vi "String Destroy.vi"(8 "error in (no error)":errorcluster, 11 "String DVR in":refnum<data-value>) -> (0 "error out":errorcluster)   [LabVIEW 2010, in "MDSplus.lvlib"]
uses:
  <vilib>/MDSplus/Library/MDSplus.lvlib
  <vilib>/MDSplus/Classes/Data_Class/Scalar_Class/String_Class/String.lvclass
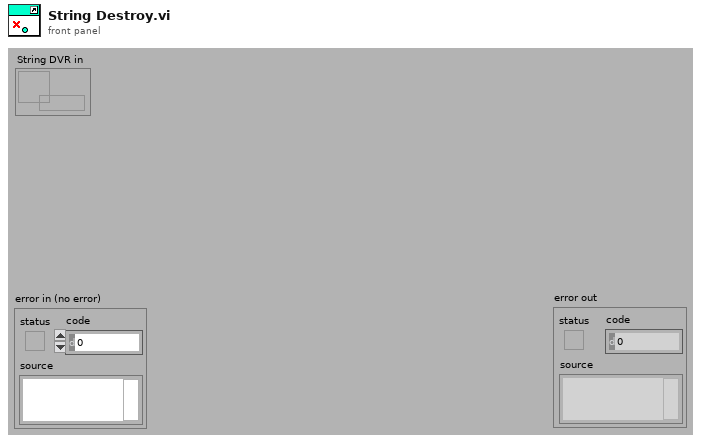
[diagram p1: front panel]
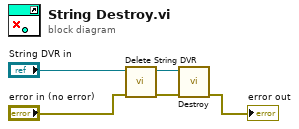
[diagram p0: block diagram]
diagram:
  n1 = call <vilib>:"Delete String DVR.vi"("error in (no error)"="error in (no error)", "String DVR in"="String DVR in") -> ("error out"=w2:errorcluster, "String out"=w3:refnum<class "String.lvclass">)  [unwired: 8 in]
  n2 = call-dynamic "Destroy.vi"("error in (no error)"=w2, "String in"=w3) -> ("error out"=→"error out":errorcluster)  [unwired: 9 in]
